vi "ImagTest.vi"() -> ()   [LabVIEW 2014]
panel:
  in  "Color Palette":cluster{"Red":u8, "Green":u8, "Blue":u8}[](array[cluster])
  in  "TIFF Options":T1={"Rows Per Strip"=0, "Photometric"=1, "Compression Type"=0} {"Compression Type" items=["None", "JPEG", "Run Length Encoded", "Zip"]; "Photometric" items=["WhiteIsZero", "BlackIsZero"]}
  in  "X Resolution":i32
  in  "Y Resolution":i32
  out "error out":errorcluster
  out "Image":T2(plugin-control)
  out "Array":u16[][](array[numeric])
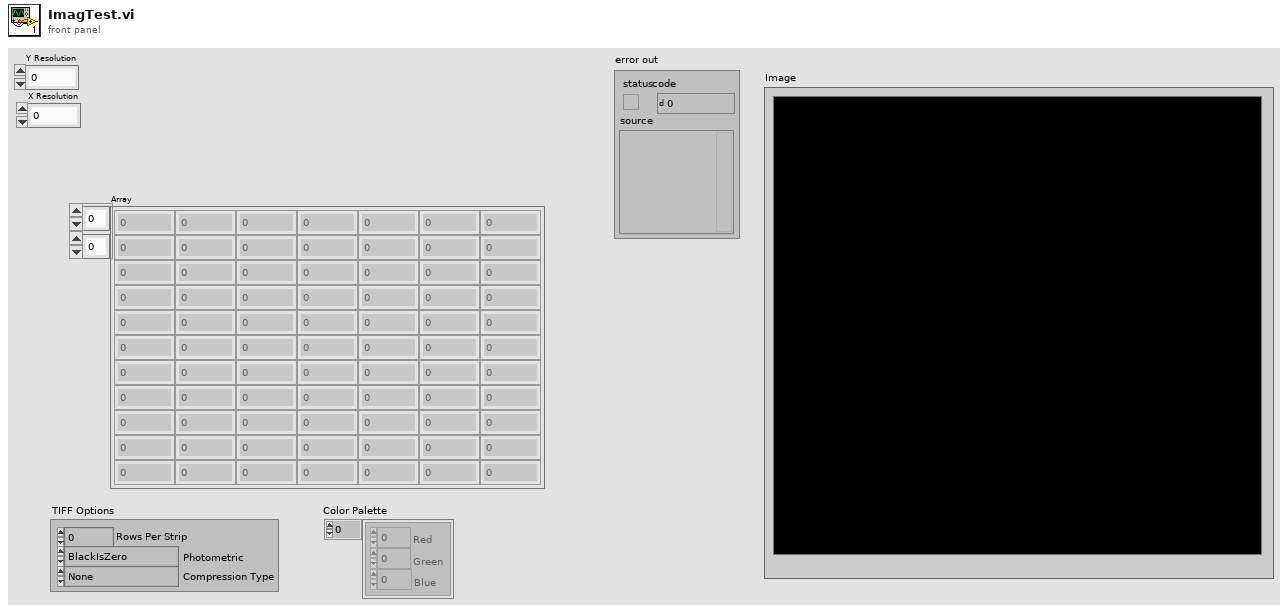
[diagram p1: front panel]
types:
  T1 = cluster{"Rows Per Strip":i32, "Photometric":i32, "Compression Type":i32}
  T2 = typedef "IMAQ Image.ctl" = refnum<image>
  T3 = typedef "Image Type" = u32
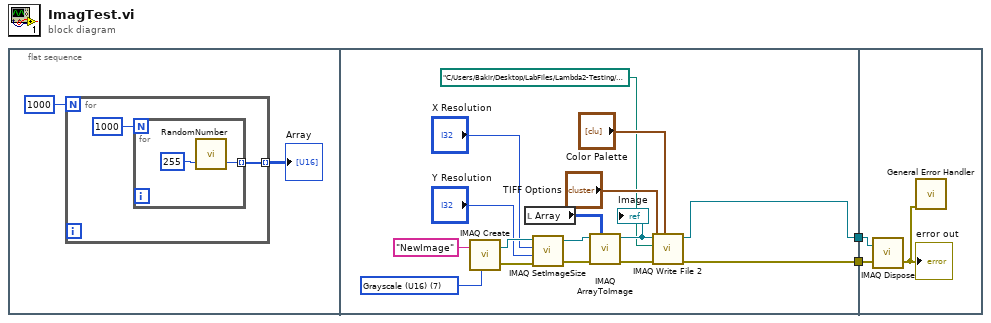
[diagram p0: block diagram]
diagram:
  n1 = flat-sequence {
    tunnel: [w9] -> w2
    tunnel: [w10] -> w1
    tunnel: w2 -> [w27]
    tunnel: w1 -> [w26]
    frame #0 {
      n2 = for {
        N: 1000 -> [_]
        tunnel: [w6] -> w4 mode=indexing
        n3 = for {
          N: 1000 -> [_]
          tunnel: [w7] -> w6 mode=indexing
          n4 = call <vilib>:"RandomNumber.vi"("Max Value"=255) -> ("Random Number"=w7:u16)  [unwired: 2 in, 1 out]
        }
      }
      "Array" <- w4
    }
    frame #1 {
      w23 = T3 7 items=["Grayscale (U8)", "Grayscale (I16)", "Grayscale (SGL)", "Complex (CSG)", "RGB (U32)", "HSL (U32)", "RGB (U64)", "Grayscale (U16)"] ("Image Type")
      n5 = call "IMAQ Create"("Image Name"="NewImage", "Image Type"=w23) -> ("New Image"=w16:T2, "error out"=w18:errorcluster)  [unwired: 3 in]
      n6 = local read "Array"() -> (w22:u16[][])
      n7 = call "IMAQ SetImageSize"("error in (no error)"=w18, "Y Resolution"="Y Resolution", "X Resolution"="X Resolution", "Image"=w16) -> ("error out"=w19:errorcluster, "Image Out"=w17:T2)  [unwired: 1 in]
      n8 = call "IMAQ ArrayToImage"("Image Pixels (U16)"=w22, "error in (no error)"=w19, "Image"=w17) -> ("error out"=w20:errorcluster, "Image Out"=w21:T2)  [unwired: 7 in]
      "Image" <- w21
      n9 = call-poly "IMAQ Write File 2"("Color Palette"="Color Palette", "error in (no error)"=w20, "TIFF Options"="TIFF Options", "File Path"=path "C:/Users/Bakir/Desktop/LabFiles/Lambda2-Testing/NewImage.tiff", "Image"=w21) -> ("error out"=w9:errorcluster, "Image Out (duplicate)"=w10:T2)  [unwired: 5 in]
    }
    frame #2 {
      n10 = call "IMAQ Dispose"("Image"=w26, "error in (no error)"=w27) -> ("error out"=w25:errorcluster)  [unwired: 4 in]
      "error out" <- w25
      n11 = call <vilib>:"General Error Handler.vi"("error in (no error)"=w25) -> ()  [unwired: 10 in, 5 out]
    }
  }
